vi "HapticSPM_force_bonding_3D.vi"() -> ()   [LabVIEW 2023]
uses:
  Haptic-Programming-Interface/LabVIEW VIs/Haptic Prog Interface/Haptic Prog Interface.lvlib
panel:
  out "Position":T1 {"z (mm)" format="%.1f"; "y (mm)" format="%.1f"; "x (mm)" format="%.1f"}
  out "Stylus":refnum<vi>(3d-picture)
  out "k":dbl format="%#_13g"
  out "Setpoint":dbl format="%#_13g"
  out "Force Function":string
  in  "Input Function":i32 min=0 max=2 step=1
  out "Force vs Distance":cluster{dbl[], dbl[]}(graph)
  out "Force":dbl(knob) scale=0.0..4.0
  in  "Gain":dbl=1.0 caption="Numeric" format="%.1g"
  # "Super Ultra Mega Haptic SPM Controller 3000"
  # "Move pen in all three dimensions to calibrate before feeling surface\n\nUse the \"PAGE UP\" or \"PAGE DOWN\" key to change the force function\n\nHold the pen as high as possible before changing force functions"
  # "Force"
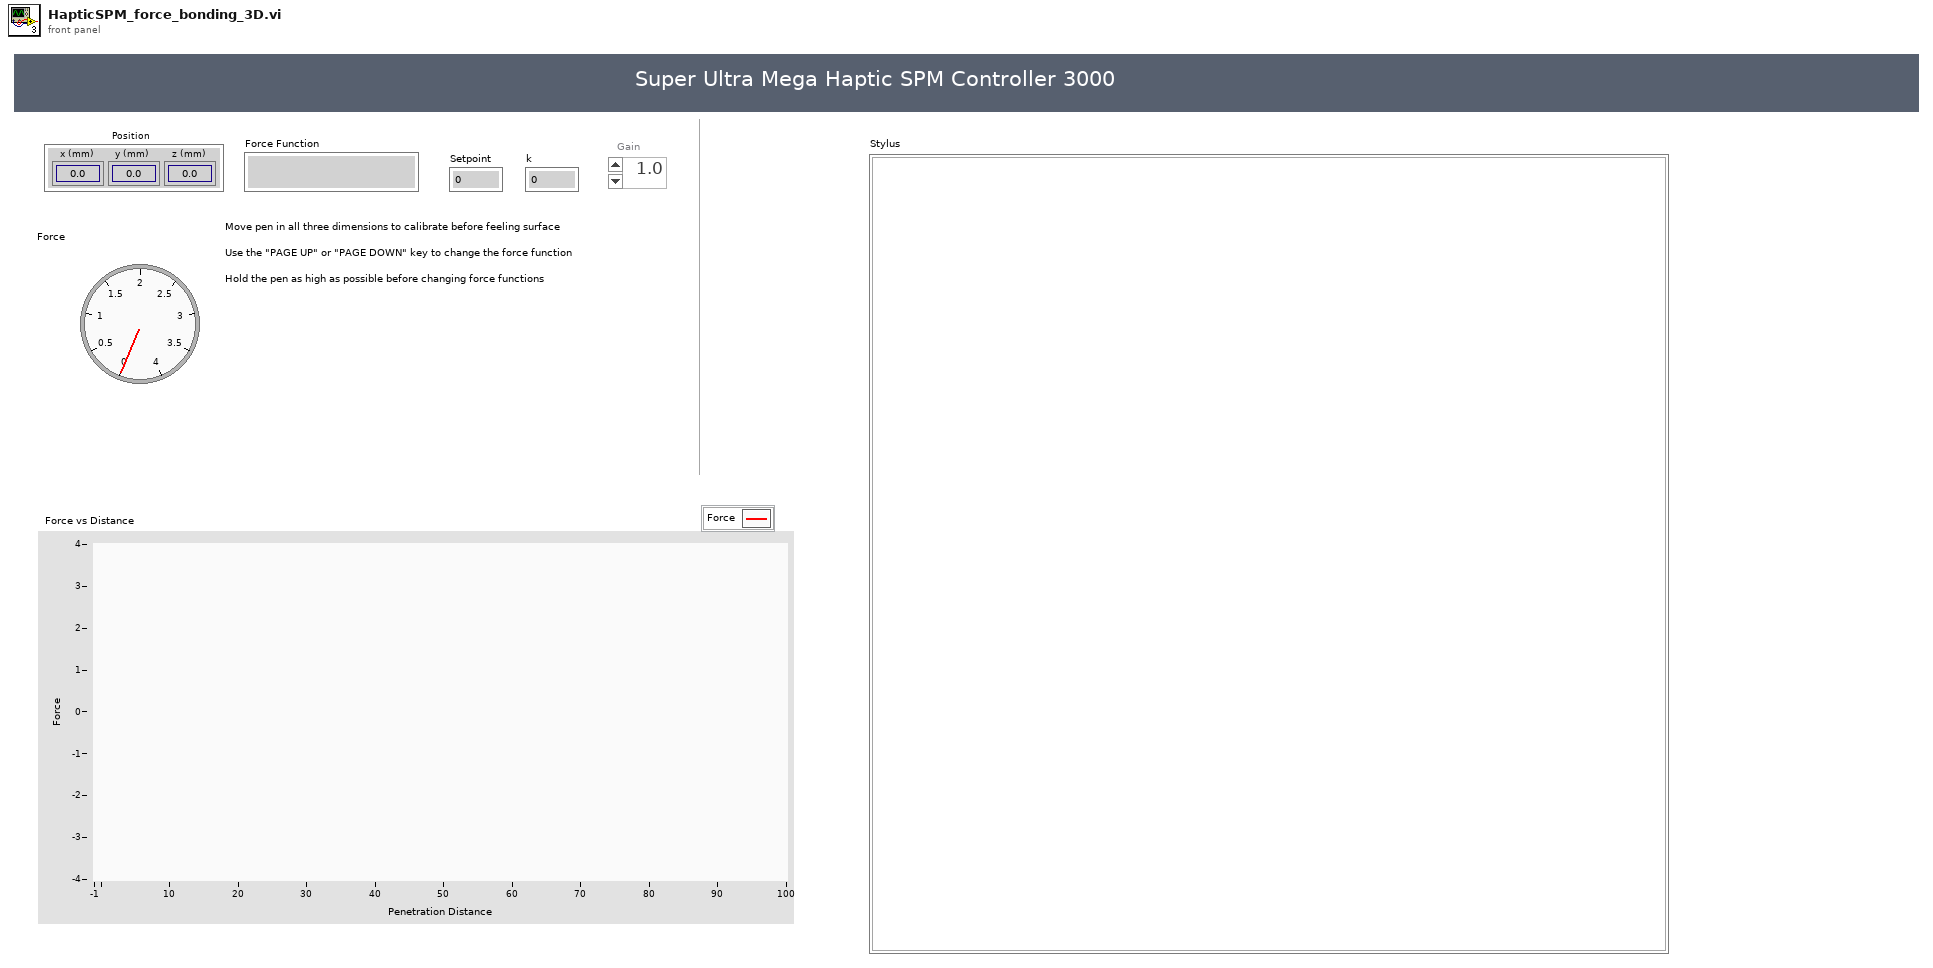
[diagram p1: front panel]
types:
  T1 = cluster{"x (mm)":dbl, "y (mm)":dbl, "z (mm)":dbl}
  T2 = cluster{"Fx (N)":dbl, "Fy (N)":dbl, "Fz (N)":dbl}
  T3 = cluster{"kx (N/m)":dbl, "ky (N/m)":dbl, "kz (N/m)":dbl}
  T4 = cluster{"X Drag":bool, "Y Drag":bool, "Z Drag":bool}
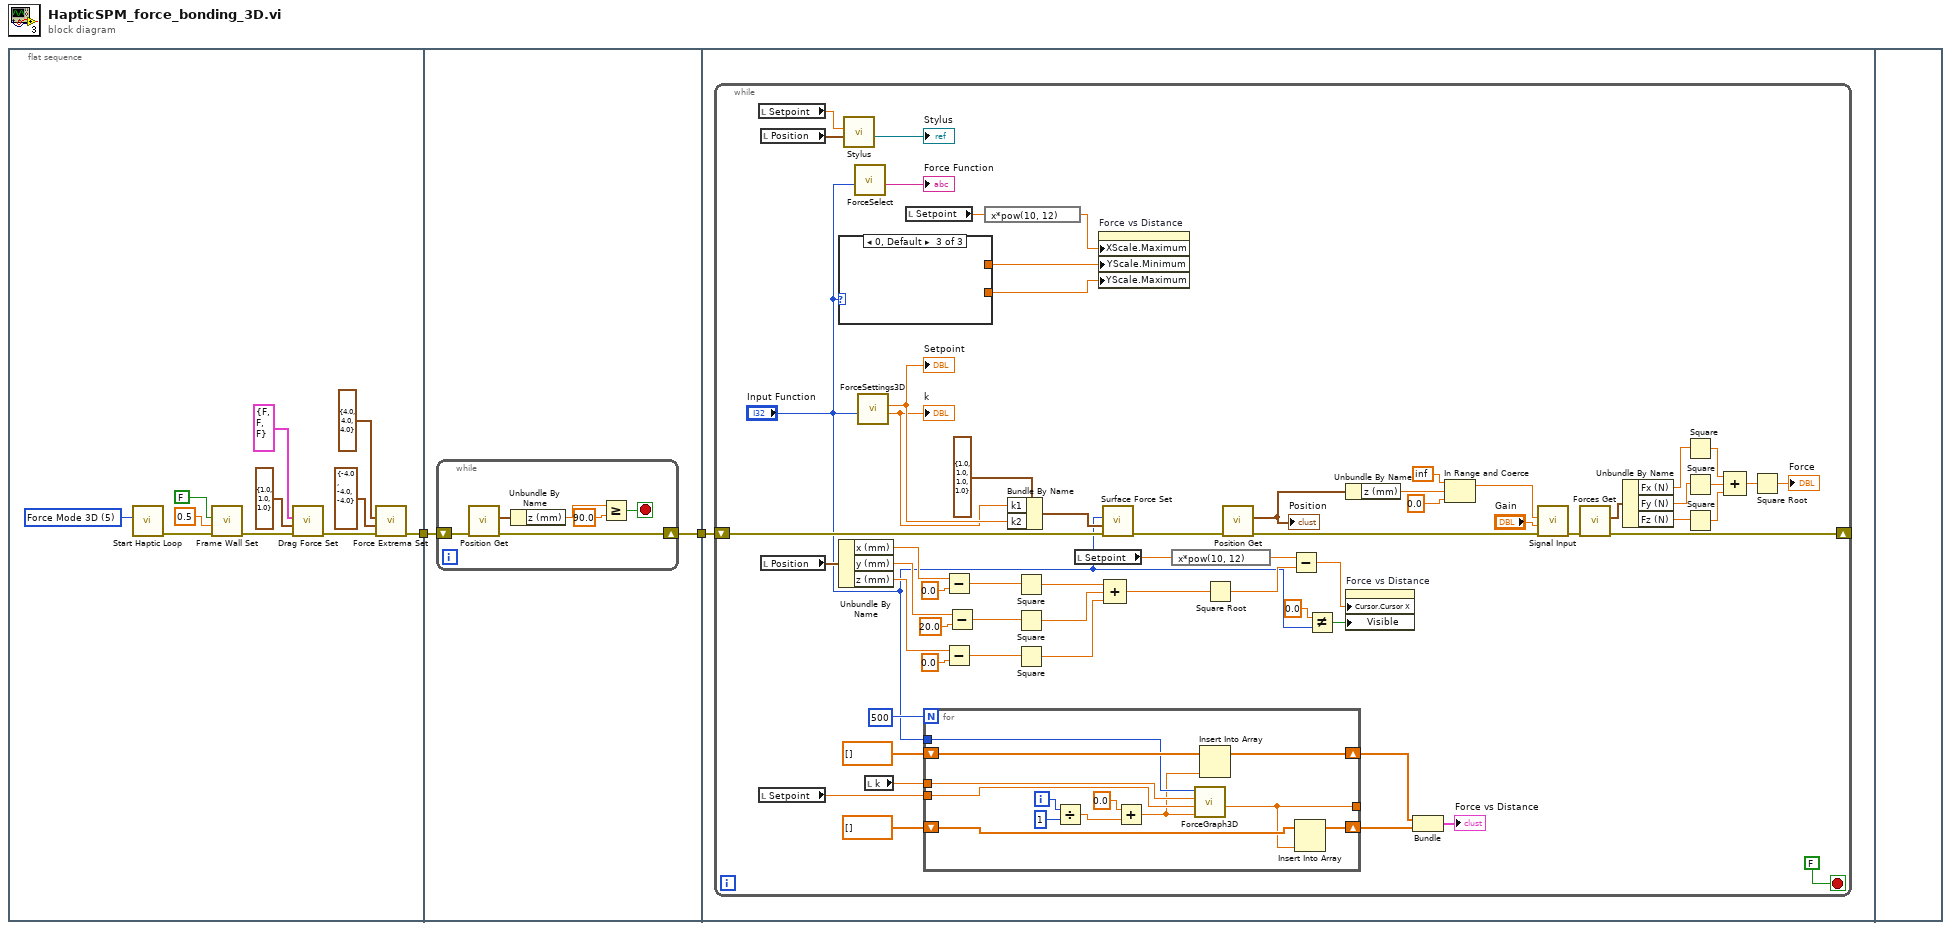
[diagram p0: block diagram]
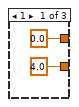
[diagram p2: hidden frame]
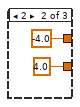
[diagram p3: hidden frame]
diagram:
  n1 = flat-sequence {
    tunnel: [w11] -> w2
    tunnel: w2 -> [w15]
    tunnel: [w14] -> w1
    tunnel: w1 -> [w22]
    frame #0 {
      w13 = u16 5 items=["Custom Mode", "Read Mode", "Write Mode", "Position Mode", "Force Mode 1D", "Force Mode 3D"] ("Mode Selection")
      n2 = call "Start Haptic Loop.vi"("Mode Selection"=w13) -> ("error out"=w4:errorcluster)  [unwired: 10 in]
      n3 = call "Frame Wall Set.vi"("error in (no error)"=w4, "Wall Stiffness (N/m)"=0.5 ("Wall Stiffness"), "Restrict to Frame"=FALSE) -> ("error out"=w3:errorcluster)  [unwired: 8 in]
      n4 = call "Drag Force Set.vi"("error in (no error)"=w3, "Drag Coefficients (N/m)"=T3 {"kx (N/m)"=1.0, "ky (N/m)"=1.0, "kz (N/m)"=1.0} ("Drag Coefficients"), "Drag Force Toggles"=T4 {"X Drag"=FALSE, "Y Drag"=FALSE, "Z Drag"=FALSE}) -> ("error out"=w12:errorcluster)  [unwired: 8 in]
      n5 = call "Force Extrema Set.vi"("error in (no error)"=w12, "Minimum Force (N)"=T2 {"Fx (N)"=-4.0, "Fy (N)"=-4.0, "Fz (N)"=-4.0} ("Minimum Force"), "Maximum Force (N)"=T2 {"Fx (N)"=4.0, "Fy (N)"=4.0, "Fz (N)"=4.0} ("Maximum Force")) -> ("error out"=w11:errorcluster)  [unwired: 8 in]
    }
    frame #1 {
      n6 = while {
        shift-right: [w20] -> w14
        shift-left: w15 -> [w21]
        stop <- w16 stop-if-true
        n7 = call "Position Get.vi"("error in (no error)"=w21) -> ("error out"=w20:errorcluster, "Position"=w19:T1)  [unwired: 9 in]
        n8 = Unbundle By Name(w19) -> ("z (mm)"=w18:dbl)
        n9 = Greater Or Equal?(x=w18, y=90.0) -> (x >= y?=w16:bool)
      }
    }
    frame #2 {
      n10 = while {
        shift-right: [w70] -> _
        shift-left: w22 -> [w84]
        stop <- FALSE ("Boolean") stop-if-true
        n11 = local read "Setpoint"() -> (w57:dbl)
        n12 = local read "Setpoint"() -> (w71:dbl)
        n13 = local read "Position"() -> (w59:T1)
        n14 = local read "Position"() -> (w55:T1)
        n15 = case shown="0, Default" "Input Function" {
          tunnel: [0.0 ("YScale.Minimum") -4.0 ("YScale.Minimum") _] -> w32
          tunnel: [4.0 ("YScale.Maximum") 4.0 ("YScale.Maximum") _] -> w31
          frame 1 {
          }
          frame 2 {
          }
          frame 0, Default {
          }
        }
        n16 = Unbundle By Name(w55) -> ("x (mm)"=w52:dbl, "y (mm)"=w51:dbl, "z (mm)"=w50:dbl)
        n17 = call "Stylus.vi"("Position"=w59, "Radius"=w57) -> ("3D Picture"=→"Stylus":refnum<vi>)  [unwired: 8 in, 1 out]
        n18 = call "ForceSelect.vi"("Input Function"="Input Function") -> ("Force Function"=→"Force Function":string)  [unwired: 10 in]
        n19 = call "ForceSettings3D.vi"("Function"="Input Function") -> ("k"=w61:dbl, "Setpoint"=w62:dbl)  [unwired: 9 in]
        "Setpoint" <- w62
        "k" <- w61
        n20 = local read "k"() -> (w72:dbl)
        n21 = local read "Setpoint"() -> (w35:dbl)
        n22 = for {
          N: 500 -> [_]
          shift-right: [w101] -> w77
          shift-left: dbl[] [] -> [w99]
          shift-right: [w100] -> w78
          shift-left: dbl[] [] -> [w98]
          tunnel: "Input Function" -> [w94]
          tunnel: [w97] -> _
          tunnel: w71 -> [w96]
          tunnel: w72 -> [w95]
          i -> [w92]
          n23 = Divide(x=w92, y=1) -> (x/y=w91:dbl)
          n24 = Add(x=0.0, y=w91) -> (x+y=w89:dbl)
          n25 = call "ForceGraph3D.vi"("number"=w89, "Setpoint"=w96, "k"=w95, "Function"=w94) -> ("force"=w97:dbl)  [unwired: 7 in]
          n26 = Insert Into Array(array=w98, new element=w89) -> (w100:dbl[])  [unwired: 1 in]
          n27 = Insert Into Array(array=w99, new element=w97) -> (w101:dbl[])  [unwired: 1 in]
        }
        n28 = Subtract(x=w52, y=0.0) -> (x-y=w46:dbl)
        n29 = Subtract(x=w50, y=0.0) -> (x-y=w44:dbl)
        n30 = Subtract(x=w51, y=20.0) -> (x-y=w45:dbl)
        n31 = expression code="x*pow(10, 12)"(w35) -> (w34:dbl)
        n32 = Bundle By Name(cluster=cluster{"k1":dbl, "k2":dbl, "k3":dbl, "k4":dbl} {"k1"=1.0, "k2"=1.0, "k3"=1.0, "k4"=1.0} ("Force Constants"), "k1"=w61, "k2"=w62) -> (w80:cluster{"k1":dbl, "k2":dbl, "k3":dbl, "k4":dbl})
        n33 = Square(x=w46) -> (x^2=w43:dbl)
        n34 = Square(x=w45) -> (x^2=w42:dbl)
        n35 = Square(x=w44) -> (x^2=w41:dbl)
        n36 = local read "Setpoint"() -> (w48:dbl)
        n37 = property on="Force vs Distance" class="XYGraph (strict)"("XScale.Maximum"=w34, "YScale.Minimum"=w32, "YScale.Maximum"=w31) -> ()  [unwired: 2 in, 2 out]
        n38 = call "Surface Force Set.vi"("error in (no error)"=w84, "Force Constants"=w80, "Force Settings"="Input Function") -> ("error out"=w67:errorcluster)  [unwired: 8 in]
        n39 = Compound Arithmetic op=ADD(w43, w42, w41) -> (w49:dbl)
        n40 = expression code="x*pow(10, 12)"(w48) -> (w40:dbl)
        n41 = Square Root(x=w49) -> (sqrt(x)=w47:dbl)
        n42 = call "Position Get.vi"("error in (no error)"=w67) -> ("error out"=w66:errorcluster, "Position"=w58:T1)  [unwired: 9 in]
        "Position" <- w58
        n43 = Subtract(x=w40, y=w47) -> (x-y=w39:dbl)
        n44 = Not Equal?(x=0.0, y="Input Function") -> (x != y?=w54:bool)
        n45 = Unbundle By Name(w58) -> ("z (mm)"=w65:dbl)
        n46 = property on="Force vs Distance" class="XYGraph (strict)"("Cursor.Cursor X"=w39, "Visible"=w54) -> ()  [unwired: 2 in, 2 out]
        n47 = Bundle(w78, w77) -> (→"Force vs Distance":cluster{dbl[], dbl[]})  [unwired: 1 in]
        n48 = In Range and Coerce(upper limit=inf, x=w65, lower limit=0.0) -> (coerced(x)=w56:dbl)  [unwired: 1 out]
        n49 = call "Signal Input.vi"("error in (no error)"=w66, "Gain"="Gain", "Signal"=w56) -> ("error out"=w83:errorcluster)  [unwired: 8 in]
        n50 = call "Forces Get.vi"("error in (no error)"=w83) -> ("error out"=w70:errorcluster, "Force (N)"=w79:T2)  [unwired: 9 in]
        n51 = Unbundle By Name(w79) -> ("Fx (N)"=w30:dbl, "Fy (N)"=w29:dbl, "Fz (N)"=w28:dbl)
        n52 = Square(x=w30) -> (x^2=w27:dbl)
        n53 = Square(x=w29) -> (x^2=w26:dbl)
        n54 = Square(x=w28) -> (x^2=w25:dbl)
        n55 = Compound Arithmetic op=ADD(w27, w26, w25) -> (w24:dbl)
        n56 = Square Root(x=w24) -> (sqrt(x)=→"Force":dbl)
      }
    }
    frame #3 {
    }
  }
